vi "Shift Coordinate by Direction.vi"(6 "Direction":T1, 10 "X in":i32, 11 "Y in":i32) -> (2 "X out":i32, 3 "Y out":i32)   [LabVIEW 2017, in "Uno.lvclass"]
uses:
  Uno.lvclass
  Type Defs/Direction Enum.ctl
  Type Defs/SB Type Defs.lvlib
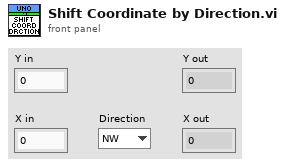
[diagram p1: front panel]
types:
  T1 = typedef "SB Type Defs.lvlib/Direction Enum.ctl" = enum16{"NW", "N", "NE", "E", "SE", "S", "SW", "W"}
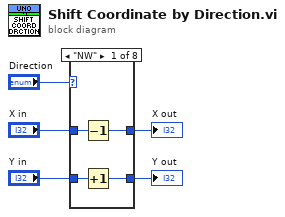
[diagram p0: block diagram]
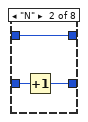
[diagram p2: hidden frame]
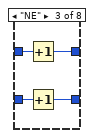
[diagram p3: hidden frame]
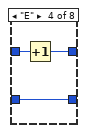
[diagram p4: hidden frame]
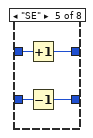
[diagram p5: hidden frame]
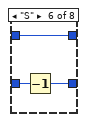
[diagram p6: hidden frame]
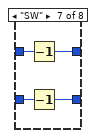
[diagram p7: hidden frame]
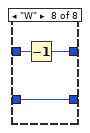
[diagram p8: hidden frame]
diagram:
  n1 = case shown="\"NW\"" "Direction" {
    tunnel: "Y in" -> [w9 w12 w16 w18 w23 w26 w30 w32]
    tunnel: "X in" -> [w8 w10 w15 w19 w22 w24 w29 w33]
    tunnel: [w7 w11 w14 w18 w21 w25 w28 w32] -> w3
    tunnel: [w6 w10 w13 w17 w20 w24 w27 w31] -> w4
    frame "NW" {
      n2 = Decrement(x=w8) -> (x-1=w6:i32)
      n3 = Increment(x=w9) -> (x+1=w7:i32)
    }
    frame "N" {
      n4 = Increment(x=w12) -> (x+1=w11:i32)
    }
    frame "NE" {
      n5 = Increment(x=w15) -> (x+1=w13:i32)
      n6 = Increment(x=w16) -> (x+1=w14:i32)
    }
    frame "E" {
      n7 = Increment(x=w19) -> (x+1=w17:i32)
    }
    frame "SE" {
      n8 = Increment(x=w22) -> (x+1=w20:i32)
      n9 = Decrement(x=w23) -> (x-1=w21:i32)
    }
    frame "S" {
      n10 = Decrement(x=w26) -> (x-1=w25:i32)
    }
    frame "SW" {
      n11 = Decrement(x=w29) -> (x-1=w27:i32)
      n12 = Decrement(x=w30) -> (x-1=w28:i32)
    }
    frame "W" {
      n13 = Decrement(x=w33) -> (x-1=w31:i32)
    }
  }
  "X out" <- w4
  "Y out" <- w3
